vi "state_to_complex.vi"(11 "KF in":T1 {"K" format="%#_3g"; "y lim" format="%#_3g"; "x lim" format="%#_3g"; "P" format="%#_3g"; "H" format="%#_3g"; "x" format="%#_3g"; "Q" format="%#_3g"; "R" format="%#_3g"; "B" format="%#_3g"; "A" format="%#_3g"}) -> (3 "Amplitudes":cdb[](array[numeric]))   [LabVIEW 2014]
uses:
  utilities/labview/kalman_filter.ctl
  <vilib>/Analysis/Matrix/Datatypes/RealMatrix.ctl
  <vilib>/Analysis/Matrix/NI_Matrix.lvlib
panel:
  # "Kalman filter is currently single state (signal amplitude), with 6x blocking (1x6 matrix).: \n    [x real, x imag, y real, y imag, z real, z imag]"
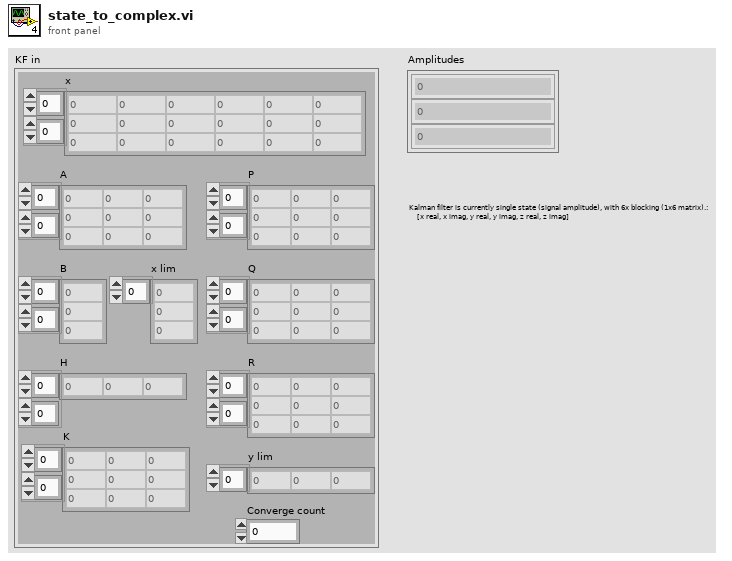
[diagram p1: front panel]
types:
  T1 = typedef "kalman_filter.ctl" = cluster{"A":T2, "B":T2, "H":T2, "Q":T2, "R":T2, "x":T2, "P":T2, "x lim":dbl[], "y lim":dbl[], "K":T2, "Converge count":i32}
  T2 = typedef "NI_Matrix.lvlib/RealMatrix.ctl" = dbl[][]
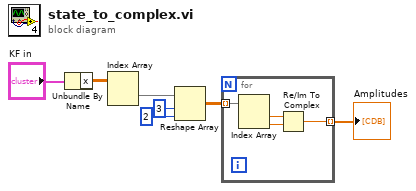
[diagram p0: block diagram]
diagram:
  n1 = Unbundle By Name("KF in") -> ("x"=w7:T2)
  n2 = Index Array(array=w7) -> (element=w5:dbl[])  [unwired: 2 in]
  n3 = Reshape Array(w5, 3 ("dimension size"), 2 ("dimension size")) -> (w2:dbl[][])
  n4 = for {
    tunnel: w2 -> [w9] mode=indexing
    tunnel: [w8] -> w1 mode=indexing
    n5 = Index Array(array=w9) -> (element #1=w10:dbl, element #2=w11:dbl)  [unwired: 2 in]
    n6 = Re/Im To Complex(1:w11, 2:w10) -> (0:w8:cdb)
  }
  "Amplitudes" <- w1
